vi "Calculate Efficiency.vi"(8 "load current measurements":dbl, 9 "load voltage measurements":dbl, 10 "source current measurements":dbl, 11 "source voltage measurements":dbl) -> (3 "Efficiency(%)":dbl)   [LabVIEW 2025, in "Scalar Efficiency And Load Regulation_PMIC.lvlib"]
uses:
  Scalar Efficiency And Load Regulation_PMIC.lvlib
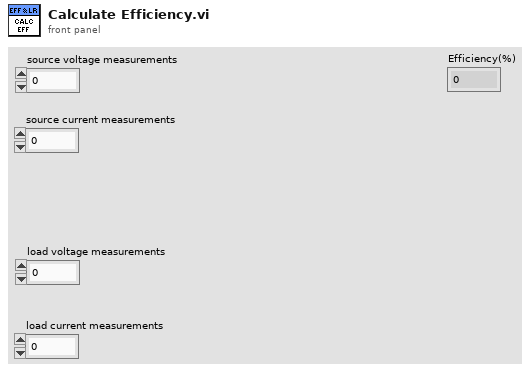
[diagram p1: front panel]
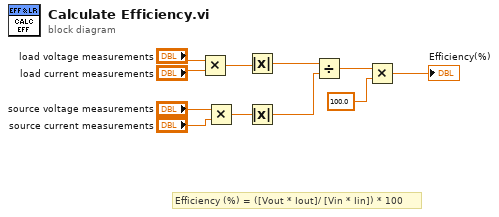
[diagram p0: block diagram]
diagram:
  # "Efficiency (%) = ([Vout * Iout]/ [Vin * Iin]) * 100"
  n1 = Multiply(x="load voltage measurements", y="load current measurements") -> (x*y=w6:dbl)
  n2 = Multiply(x="source voltage measurements", y="source current measurements") -> (x*y=w5:dbl)
  n3 = Absolute Value(x=w6) -> (abs(x)=w11:dbl)
  n4 = Absolute Value(x=w5) -> (abs(x)=w10:dbl)
  n5 = Divide(x=w11, y=w10) -> (x/y=w9:dbl)
  n6 = Multiply(x=w9, y=100.0) -> (x*y=→"Efficiency(%)":dbl)
